vi "StringToString.vi"(1 "String":string) -> (0 "Output":string)   [LabVIEW 2020]
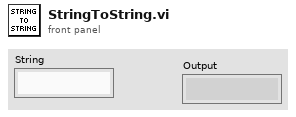
[diagram p1: front panel]
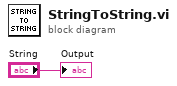
[diagram p0: block diagram]
diagram:
  "Output" <- "String"
